vi "Bispectrum Analysis.vi"() -> ()   [LabVIEW 2023]
doc: "This example shows how to compute the bispectrum of a univariate time series using the TSA Bispectrum VI, and plot the bispectrum with 3D plot control.\n\n<b>Instructions:</b>\n1) Run this VI.\n2) Try different methods and settings.\n3) Observe the bispectrum of the EEG signal."
uses:
  <vilib>/Native 3D Graph/xcontrol/3DPC_SurfacePlot.xctl
  <vilib>/addons/Time Series Analysis/Utilities.llb/TSA Data.ctl
  <vilib>/addons/Time Series Analysis/Correlation and Spectral Analysis.llb/TSA Bispectrum (Waveform).vi
  <vilib>/addons/_Advanced Signal Processing/NI_AdvSigProcTSA.lvlib
panel:
  in  "Method 2":enum32{"FFT", "AR Model"}(tab)
  in  "Window info":T1={"Window"=1, "Length"=100, "Overlap (%)"=90.0} {"Window" items=["None ", "Hanning", "Hamming", "Blackman-Harris", "Exact Blackman", "Blackman", "Flat Top", "4 Term B-Harris ", "7 Term B-Harris", "Low Sidelobe"]}
  in  "AR setting":cluster{"Method":u16, "AR Order":i32}={"Method"=0, "AR Order"=4} {"Method" items=["Forward-Backward", "Least-Squares", "Yule-Walker", "Burg-Lattice", "Geometric-Lattice"]}
  out "averaging done?":bool
  in  "Averaging Parameters":T2={"Averaging Mode"=0, "Weighting Mode"=1, "Number of Averages"=10} {"Number of Averages" min=1; "Weighting Mode" items=["Linear", "Exponential"]; "Averaging Mode" items=["No Averaging", "Vector Averaging", "RMS Averaging", "Peak Hold"]}
  out "aspt-left-top":bool
  in  "stop":bool
  in  "dB on? (F)":bool
  in  "Method":u16(ring) items=["FFT", "AR Model"]
  in  "Frequency bins":i32=256
  out "EEG":waveform(dbl)(graph)
  out "Bispectrum":refnum<class "Base Datatype.lvclass">[](xcontrol)
  # "Overview: Shows how to compute the bispectrum of a univariate time series using the TSA Bispectrum VI, and plot the bispectrum with 3D plot control.\nRequirements: LabVIEW Full Development System, Advanced Signal Processing Toolkit\nInstructions: \n1. Run this VI.\n2. Try different methods and settings.\n3. Observe the bispectrum of the EEG signal.\n4. Click Stop to stop the VI."
  # "Bispectrum Settings"
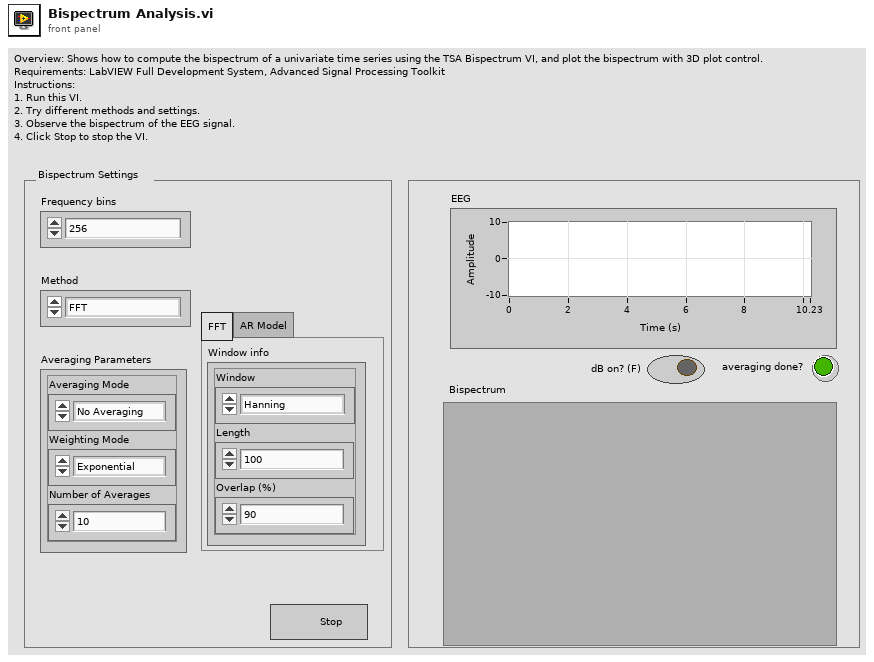
[diagram p1: front panel]
types:
  T1 = cluster{"Window":u16, "Length":i32, "Overlap (%)":dbl}
  T2 = cluster{"Averaging Mode":u16, "Weighting Mode":u16, "Number of Averages":u32}
  T3 = typedef "NI_AdvSigProcTSA.lvlib/TSA Data.ctl" = u16
  T4 = cluster{"Frequency bins":i32, "Method":u16, "Window info":cluster{"Window":u16, "Length":i32, "Overlap (%)":dbl}, "Averaging Parameters":cluster{"Averaging Mode":u16, "Weighting Mode":u16, "Number of Averages":u32}, "AR setting":cluster{"Method":u16, "AR Order":i32}}
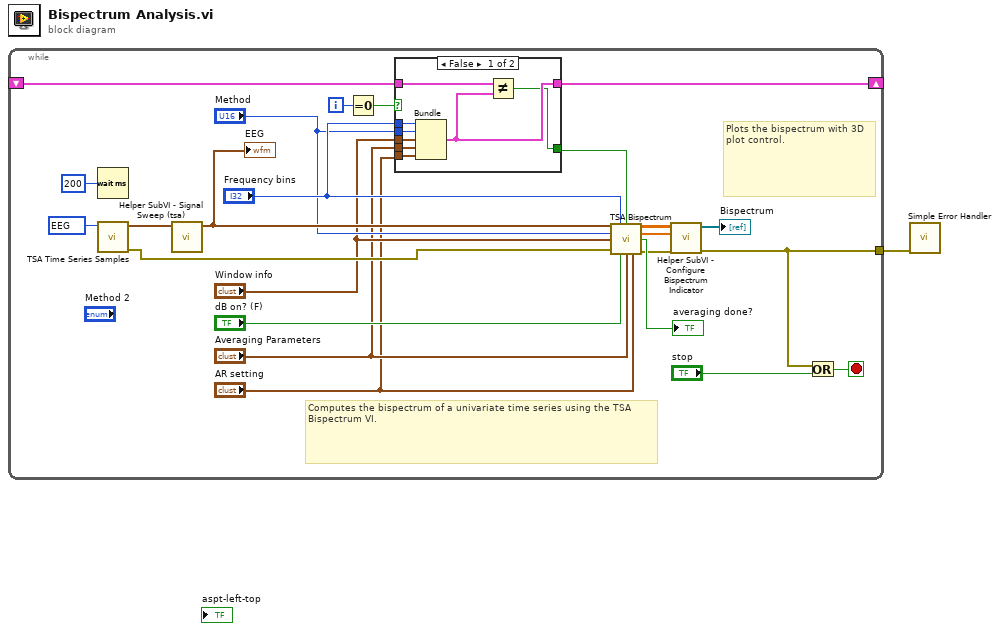
[diagram p0: block diagram]
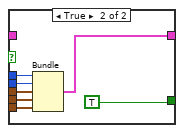
[diagram p2: hidden frame]
diagram:
  n1 = while {
    shift-right: [w9] -> _
    shift-left: _ -> [w8]
    tunnel: [w3] -> w1
    i -> [w16]
    stop <- w22 stop-if-true
    w18 = T3 210 items=["Kobe Earthquake"=201, "EEG"=210, "Bearing Vibration (simulated)"=211, "Period Product Sales"=214, "Beam Vibration (nonlinear)"=217, "Beam Vibration (linear)"=218, "Signal With Echo"=219, "Engine Knocking"=220, "Power Line"=221, "-"=200, "Beam Deflections (multivariate)"=207, "Structure Vibration (multivariate)"=208, "Human MEG (multivariate)"=222] ("data")
    # "Plots the bispectrum with 3D plot control."
    # "Computes the bispectrum of a univariate time series using the TSA Bispectrum VI."
    n2 = Wait (ms)(milliseconds to wait=u32 200 ("millisecond multiple")) -> ()  [unwired: 1 out]
    n3 = call <vilib>:"TSA Time Series Samples.vi"("data"=w18) -> ("error out"=w25:errorcluster, "univariate time series"=w20:waveform(dbl))  [unwired: 1 in, 8 out]
    n4 = call "Helper SubVI - Signal Sweep (tsa).vi"("Signal in"=w20) -> ("Signal out"=w19:waveform(dbl))  [unwired: 10 in]
    "EEG" <- w19
    n5 = Equal To 0?(x=w16) -> (x = 0?=w15:bool)
    n6 = case shown="False" w15 {
      tunnel: "Frequency bins" -> [w33 w40]
      tunnel: "Method" -> [w32 w39]
      tunnel: "Window info" -> [w31 w38]
      tunnel: "Averaging Parameters" -> [w30 w37]
      tunnel: "AR setting" -> [w29 w36]
      tunnel: [w27 w35] -> w9
      tunnel: w8 -> [w28 _]
      tunnel: [w26 TRUE] -> w7
      frame False {
        n7 = Bundle("Frequency bins"=w33, "Method"=w32, "Window info"=w31, "Averaging Parameters"=w30, "AR setting"=w29) -> (w27:T4)  [unwired: 1 in]
        n8 = Not Equal?(x=w28, y=w27) -> (x != y?=w26:bool)
      }
      frame True {
        n9 = Bundle("Frequency bins"=w40, "Method"=w39, "Window info"=w38, "Averaging Parameters"=w37, "AR setting"=w36) -> (w35:T4)  [unwired: 1 in]
      }
    }
    n10 = call-poly <vilib>:"TSA Bispectrum.vi"("Xt"=w19, "frequency bins"="Frequency bins", "initialize? (F)"=w7, "method"="Method", "window info"="Window info", "error in (no error)"=w25, "dB on? (T)"="dB on? (F)", "averaging parameters"="Averaging Parameters", "AR setting"="AR setting") -> ("S(f,f)"=w6:dbl[][], "freq bins"=w5:dbl[], "averaging done?"=→"averaging done?":bool, "error out"=w4:errorcluster)  [unwired: 2 in, 1 out]
    n11 = call "Helper SubVI - Configure Bispectrum Indicator.vi"("error in (no error)"=w4, "frequency bins"=w5, "S(f,f)"=w6) -> ("error out"=w3:errorcluster, "bispectrum  indicator"=→"Bispectrum":refnum<class "Base Datatype.lvclass">[])  [unwired: 7 in]
    n12 = Or(x=w3, y="stop") -> (x .or. y?=w22:bool)
  }
  n13 = call <vilib>:"Simple Error Handler.vi"("error in (no error)"=w1) -> ()  [unwired: 1 in, 8 out]
